vi "mod2 sub.vi"(1 "Array":i32[][](array[numeric])) -> (0 "Array 2":i32[][](array[numeric]))   [LabVIEW 2010]
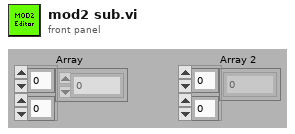
[diagram p1: front panel]
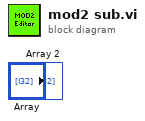
[diagram p0: block diagram]
diagram:
  "Array 2" <- "Array"
